vi "OCV Measure DC Volts.vi"(8 "error in (no error)":errorcluster, 10 "Number of Measurements":i32=128) -> (0 "error out":errorcluster, 2 "Measurements (Volts)":dbl[](array[numeric])=[3.486017932336771, 3.486017307834901, 3.486017600737179, 3.486017977248404, 3.4860177403183688, 3.4860179150120914, 3.4860177036838285, 3.4860178309889314, 3.4860177531972822, 3.486017977754826, 3.4860179330089647, 3.48601814510014, 3.486018147033395, 3.4860177431187243, 3.4860177797011875, 3.486017997042972, 3.486018038037714, 3.486017878191467, 3.486018126596086, 3.486017769724553, 3.486017992593923, 3.4860184321660705, 3.486017864938252, 3.486017411838484, 3.4860179876723802, 3.486017959684013, 3.4860179763899417, 3.4860178187665127, 3.4860181827150996, 3.486018245194682, 3.4860180098625495, 3.486017797221756, 3.4860181423306345, 3.4860176881665175, 3.486018084873098, 3.486017671108277, 3.4860178318523425, 3.4860176788045503, 3.4860177962648726, 3.4860176851712743, 3.486017790116506, 3.4860177670877572, 3.486018012605684, 3.4860178934400214, 3.486018329992307, 3.4860180981146773, 3.4860180096557576, 3.486017938785145, 3.4860183230428614, 3.4860178747798787, 3.486017814818513, 3.4860179148088757, 3.4860181999824875, 3.486017785602333, 3.486017829577085, 3.4860180105835474, 3.4860174289366563, 3.486017644862929, 3.4860178994496565, 3.4860179954448096, 3.48601793934282, 3.4860179746921376, 3.486018026188553, 3.4860175892288225, 3.4860180347614023, 3.4860181103873873, 3.4860178832560527, 3.4860180410479487, 3.486018032763997, 3.486018622537674, 3.4860181548045874, 3.486017530224023, 3.486017947248753, 3.486018043066002, 3.48601811908244, 3.4860179760940153, 3.486018418334813, 3.4860178982991576, 3.4860182376122486, 3.486017987488014, 3.486017961989586, 3.486017839712657, 3.486018154426059, 3.4860182654538283, 3.486018068682808, 3.486017939355624, 3.486018112168974, 3.486018021643548, 3.4860181301969235, 3.4860181388493037, 3.486018377605749, 3.4860181136864066, 3.4860176318841773, 3.4860180166697994, 3.4860177217403545, 3.4860181410713804, 3.4860178522251486, 3.486017813379955, 3.486018026525973, 3.4860178772425607] format="%#_9g")   [LabVIEW 2019]
doc: "This example acquires a single DC Voltage measurement. Specify the range and absolute resolution of your input signal. The measured value will be displayed in the Measurement indicator. A Boolean indicator will indicate if the measured value is out of range."
uses:
  <instrlib>/niDMM/nidmm.llb/niDMM Function.ctl
  <instrlib>/niDMM/nidmm.llb/niDMM Resolution in Digits.ctl
  <instrlib>/niDMM/nidmm.llb/niDMM Configure Measurement Digits.vi
panel:
  out "Configuration:Measurement Options:DC Noise Rejection":i32(ring)=2 items=["Auto"=-1, "Normal"=0, "Second Order"=1, "High Order"=2]
  out "Configuration:Measurement Options:ADC Calibration":i32(ring)=1 items=["Auto"=-1, "Off"=0, "On"=1]
  out "Configuration:Measurement Options:Auto Zero":i32(ring)=1 items=["Auto"=-1, "Off"=0, "On"=1, "Once"=2]
  in  "Resolution in Digits":T1=7.5 items=["3 1/2"=3.5, "4 1/2"=4.5, "5 1/2"=5.5, "6 1/2"=6.5, "7 1/2"=7.5]
  in  "Measurement Type":T2
  out "Signal Out of Range":bool
  in  "Device Name":refnum<k15>="DMM"
  in  "Range (Volts)":dbl=10.0 format="%.2p"
  # "Configuration"
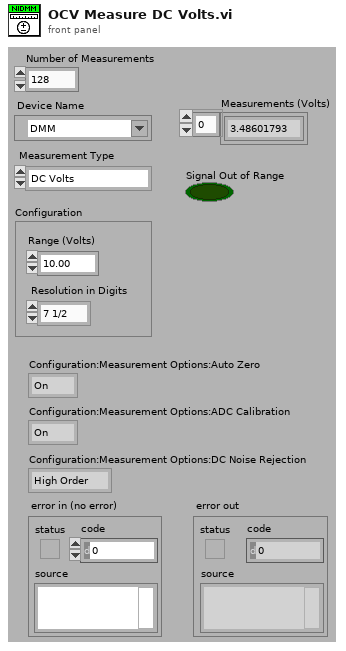
[diagram p1: front panel]
types:
  T1 = typedef "niDMM Resolution in Digits.ctl" = dbl
  T2 = typedef "niDMM Function.ctl" = enum16{"DC Volts", "AC Volts", "DC Current", "AC Current", "2-wire Resistance", "4-wire Resistance", "Diode", "Frequency", "Period", "AC Volts DC Coupled", "Capacitance", "Inductance", "Temperature"}
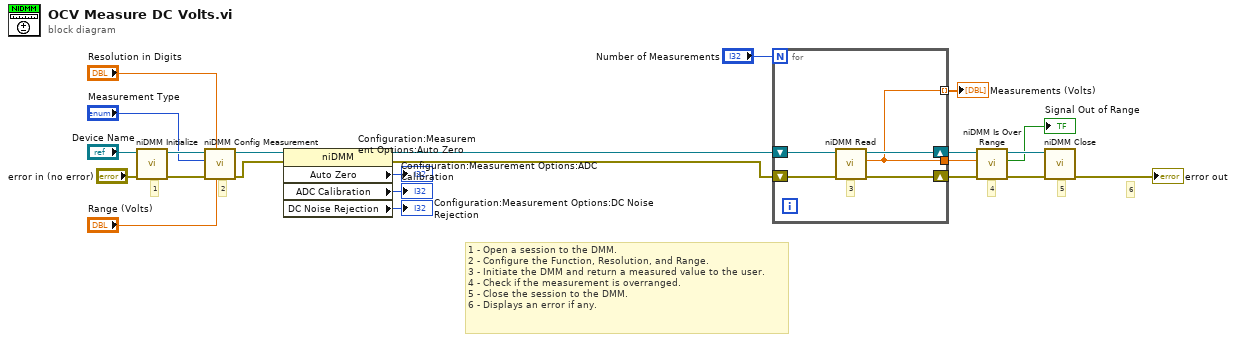
[diagram p0: block diagram]
diagram:
  # "6"
  # "1 - Open a session to the DMM.\n2 - Configure the Function, Resolution, and Range.\n3 - Initiate the DMM and return a measured value to the user.\n4 - Check if the measurement is overranged.\n5 - Close the session to the DMM.\n6 - Displays an error if any."
  # "1"
  # "5"
  # "4"
  # "2"
  n1 = call <instrlib>:"niDMM Initialize.vi"("error in (no error)"="error in (no error)", "Instrument Descriptor"="Device Name") -> ("error out"=w22:errorcluster, "instrument handle out"=w23:refnum<k15>)  [unwired: 8 in]
  n2 = call-poly <instrlib>:"niDMM Config Measurement.vi"("Range"="Range (Volts)", "Resolution in Digits"="Resolution in Digits", "error in (no error)"=w22, "Function"="Measurement Type", "instrument handle"=w23) -> ("error out"=w6:errorcluster, "instrument handle out"=w8:refnum<k15>)  [unwired: 5 in]
  n3 = property class="niDMM"(reference=w8, error in=w6) -> (reference out=w7:refnum<k15>, error out=w5:errorcluster, "Auto Zero"=→"Configuration:Measurement Options:Auto Zero":i32, "ADC Calibration"=→"Configuration:Measurement Options:ADC Calibration":i32, "DC Noise Rejection"=→"Configuration:Measurement Options:DC Noise Rejection":i32)
  n4 = for {
    N: "Number of Measurements" -> [_]
    tunnel: [w24] -> w10 mode=indexing
    shift-right: [w27] -> w17
    shift-left: w5 -> [w26]
    shift-right: [w28] -> w18
    shift-left: w7 -> [w25]
    tunnel: [w24] -> w9
    # "3"
    n5 = call <instrlib>:"niDMM Read.vi"("error in (no error)"=w26, "instrument handle"=w25) -> ("error out"=w27:errorcluster, "Measurement"=w24:dbl, "instrument handle out"=w28:refnum<k15>)  [unwired: 7 in]
  }
  "Measurements (Volts)" <- w10
  n6 = call <instrlib>:"niDMM Is Over Range.vi"("error in (no error)"=w17, "Measurement"=w9, "instrument handle"=w18) -> ("error out"=w15:errorcluster, "Over Range?"=→"Signal Out of Range":bool, "instrument handle out"=w16:refnum<k15>)  [unwired: 6 in]
  n7 = call <instrlib>:"niDMM Close.vi"("error in (no error)"=w15, "instrument handle"=w16) -> ("error out"=→"error out":errorcluster)  [unwired: 9 in]
